vi "Add Monitor Status Error.vi"(8 "error in (no error)":errorcluster, 11 "Section ref in":T1 format="%.0x") -> (0 "error out":errorcluster, 2 "Section Ptr":T1 format="%.0x", 3 "Parent Ref out":T1 format="%.0x")   [LabVIEW 2020, in "AIM ARINC 664 Scripting.lvlib"]
uses:
  AIM ARINC 664 Scripting.lvlib
  <vilib>/NI VeriStand/Custom Device API/Custom Device Item Ref.ctl
  Constants.vi
  <vilib>/NI VeriStand/Custom Device API/Custom Device API.lvlib
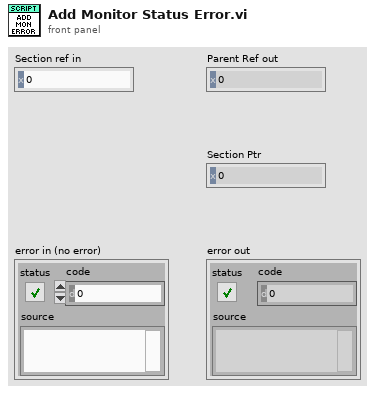
[diagram p1: front panel]
types:
  T1 = typedef "Custom Device API.lvlib/Custom Device Item Ref.ctl" = u64
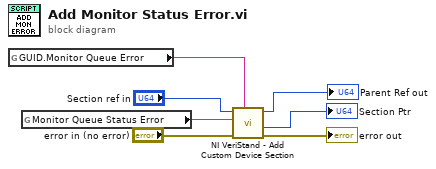
[diagram p0: block diagram]
diagram:
  n1 = global read "Constants.vi" "GUID.Monitor Queue Error"() -> (w5:string)
  n2 = global read "Constants.vi" "Monitor Queue Status Error"() -> (w3:string)
  n3 = call <vilib>:"NI VeriStand - Add Custom Device Section.vi"("GUID (Default Section)"=w5, "error in (no error)"="error in (no error)", "Section Name"=w3, "Parent Ref in"="Section ref in") -> ("error out"=→"error out":errorcluster, "Section Ptr"=→"Section Ptr":T1, "Parent Ref out"=→"Parent Ref out":T1)  [unwired: 4 in, 1 out]
